vi "draw.g.vi"(11 "midi-ui in":refnum<class "midi-ui.lvclass">) -> (2 "coordinates":cluster{"x":dbl, "y":dbl}[](array[cluster]), 3 "midi-ui out":refnum<class "midi-ui.lvclass">)   [LabVIEW 2020, in "midi-ui.lvclass"]
uses:
  midi-ui.lvclass
  midi-ui.lvclass/midi-ui.ctl
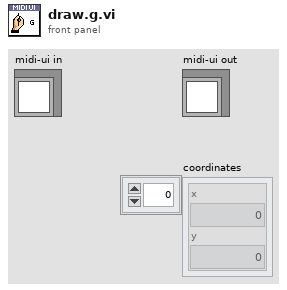
[diagram p1: front panel]
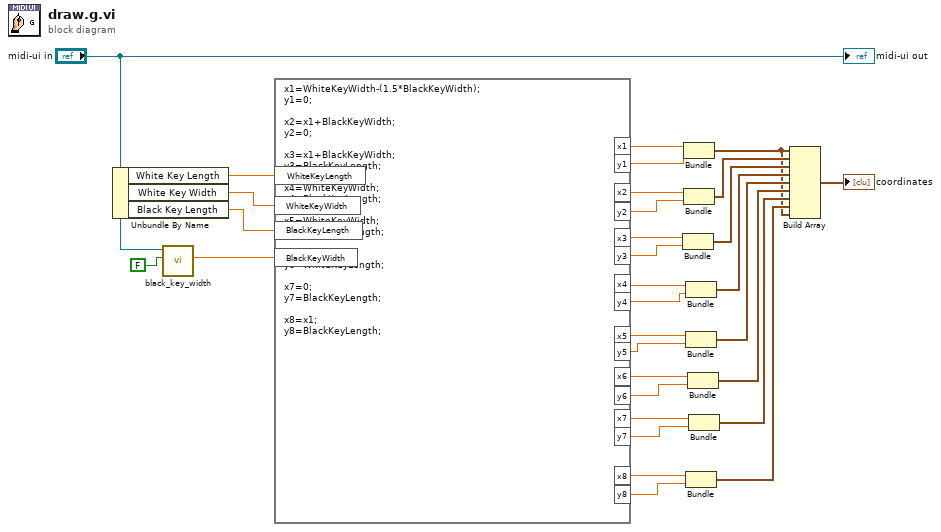
[diagram p0: block diagram]
diagram:
  n1 = Unbundle By Name("midi-ui in") -> ("White Key Length"=w4:dbl, "White Key Width"=w5:dbl, "Black Key Length"=w6:dbl)
  n2 = call "black_key_width.vi"("C# or D#?"=FALSE, "midi-ui in"="midi-ui in") -> ("Black Key Width"=w1:dbl)  [unwired: 8 in, 1 out]
  n3 = formula code="x1=WhiteKeyWidth-(1.5*BlackKeyWidth);\ny1=0;\n\nx2=x1+BlackKeyWidth;\ny2=0;\n\nx3=x1+BlackKeyWidth;\ny3=BlackKeyLength;\n\nx4=WhiteKeyWidth;\ny4=BlackKeyLength;\n\nx5=WhiteKeyWidth;\ny5=WhiteKeyLength;\n\nx6=0;\ny6=WhiteKeyLength;\n\nx7=0;\ny7=BlackKeyLength;\n\nx8=x1;\ny8=BlackKeyLength;"("WhiteKeyLength"=w4, "WhiteKeyWidth"=w5, "BlackKeyLength"=w6, "BlackKeyWidth"=w1) -> ("x1"=w31:dbl, "y1"=w30:dbl, "x2"=w18:dbl, "y2"=w19:dbl, "x3"=w20:dbl, "y3"=w29:dbl, "x4"=w21:dbl, "y4"=w22:dbl, "x6"=w23:dbl, "y6"=w24:dbl, "x7"=w25:dbl, "y7"=w26:dbl, "x8"=w27:dbl, "y8"=w28:dbl, "x5"=w10:dbl, "y5"=w11:dbl)
  n4 = Bundle("x3"=w20, "y3"=w29) -> (w16:cluster{"x3":dbl, "y3":dbl})  [unwired: 1 in]
  n5 = Bundle("x1"=w31, "y1"=w30) -> (w8:cluster{"x1":dbl, "y1":dbl})  [unwired: 1 in]
  n6 = Bundle("x2"=w18, "y2"=w19) -> (w17:cluster{"x2":dbl, "y2":dbl})  [unwired: 1 in]
  n7 = Bundle("x4"=w21, "y4"=w22) -> (w15:cluster{"x4":dbl, "y4":dbl})  [unwired: 1 in]
  n8 = Bundle("x5"=w10, "y5"=w11) -> (w9:cluster{"x5":dbl, "y5":dbl})  [unwired: 1 in]
  n9 = Bundle("x8"=w27, "y8"=w28) -> (w12:cluster{"x8":dbl, "y8":dbl})  [unwired: 1 in]
  n10 = Bundle("x6"=w23, "y6"=w24) -> (w14:cluster{"x6":dbl, "y6":dbl})  [unwired: 1 in]
  n11 = Bundle("x7"=w25, "y7"=w26) -> (w13:cluster{"x7":dbl, "y7":dbl})  [unwired: 1 in]
  n12 = Build Array(w8, w17, w16, w15, w9, w14, w13, w12, w8) -> (→"coordinates":cluster{"x1":dbl, "y1":dbl}[])
  "midi-ui out" <- "midi-ui in"
